vi "ChangeNamesDialog.vi"(10 "Device Names":string[](array[string])) -> (2 "unique names":string[](array[string]))   [LabVIEW 2013]
doc: "Present dialog to ask for unique list of device names."
panel:
  in  "OK button":bool
  # "One or more names are not unique.\nPlease give each device a unique name:"
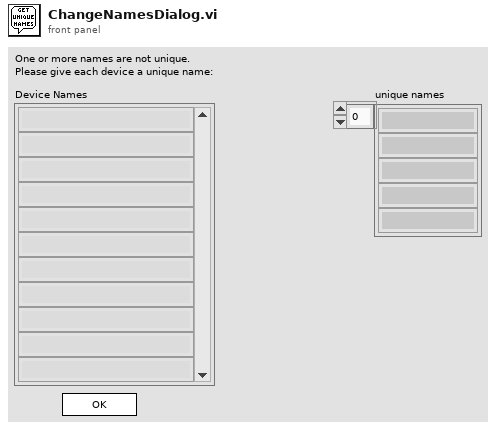
[diagram p1: front panel]
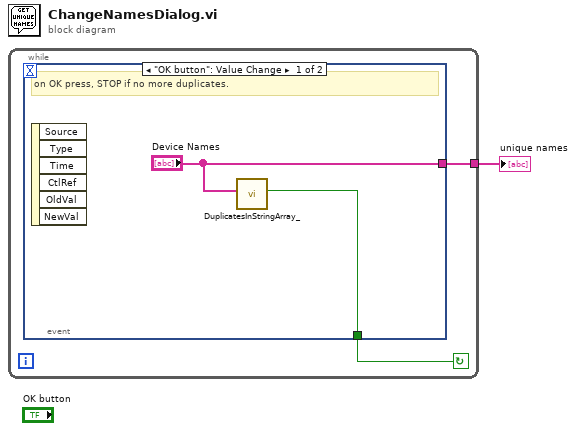
[diagram p0: block diagram]
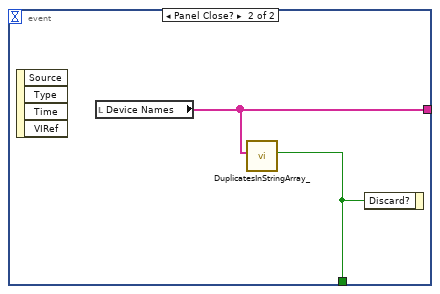
[diagram p2: hidden frame]
diagram:
  n1 = while {
    tunnel: [w3] -> w1
    stop <- w2 continue-if-true
    n2 = event shown="[0] \"OK button\": Value Change" {
      selector: _ -> [_ _]
      dyn-events: _ -> [_ _]
      timeout: _ -> [_ _]
      tunnel: ["Device Names" w7] -> w3
      tunnel: [w4 w6] -> w2
      event "OK button": Value Change {
        # "on OK press, STOP if no more duplicates."
        n3 = event-data() -> ()  [unwired: 1 in, 6 out]
        n4 = call "DuplicatesInStringArray_.vi"("String array"="Device Names") -> ("duplicates?"=w4:bool)  [unwired: 10 in]
      }
      event Panel Close? {
        n5 = event-data() -> ()  [unwired: 1 in, 4 out]
        n6 = local read "Device Names"() -> (w7:string[])
        n7 = call "DuplicatesInStringArray_.vi"("String array"=w7) -> ("duplicates?"=w6:bool)  [unwired: 10 in]
        n8 = event-data("Discard?"=w6) -> ()  [unwired: 1 in, 1 out]
      }
    }
  }
  "unique names" <- w1
